vi "AplicaPond_C_Ref_GenExterno.vi"(1 "result":string[][](array[string])) -> (0 "output array":string[][](array[string]))   [LabVIEW 2019, in "Prueba03.lvclass"]
doc: "Aplica ponderacion C a la curva de referencia hecha en Ajustes Previos 3"
uses:
  Prueba03.lvclass
panel:
  out "114db(C)":string[](array[string])
  out "94db(C)":string[](array[string])
  # "Frecuencias"
  # "94dB"
  # "114dB"
  # "94dB(A)"
  # "114dB(A)"
  # "94dB(C)"
  # "114dB(C)"
  # "94dB(Z)"
  # "114dB(Z)"
  # "Correcciones Microfono"
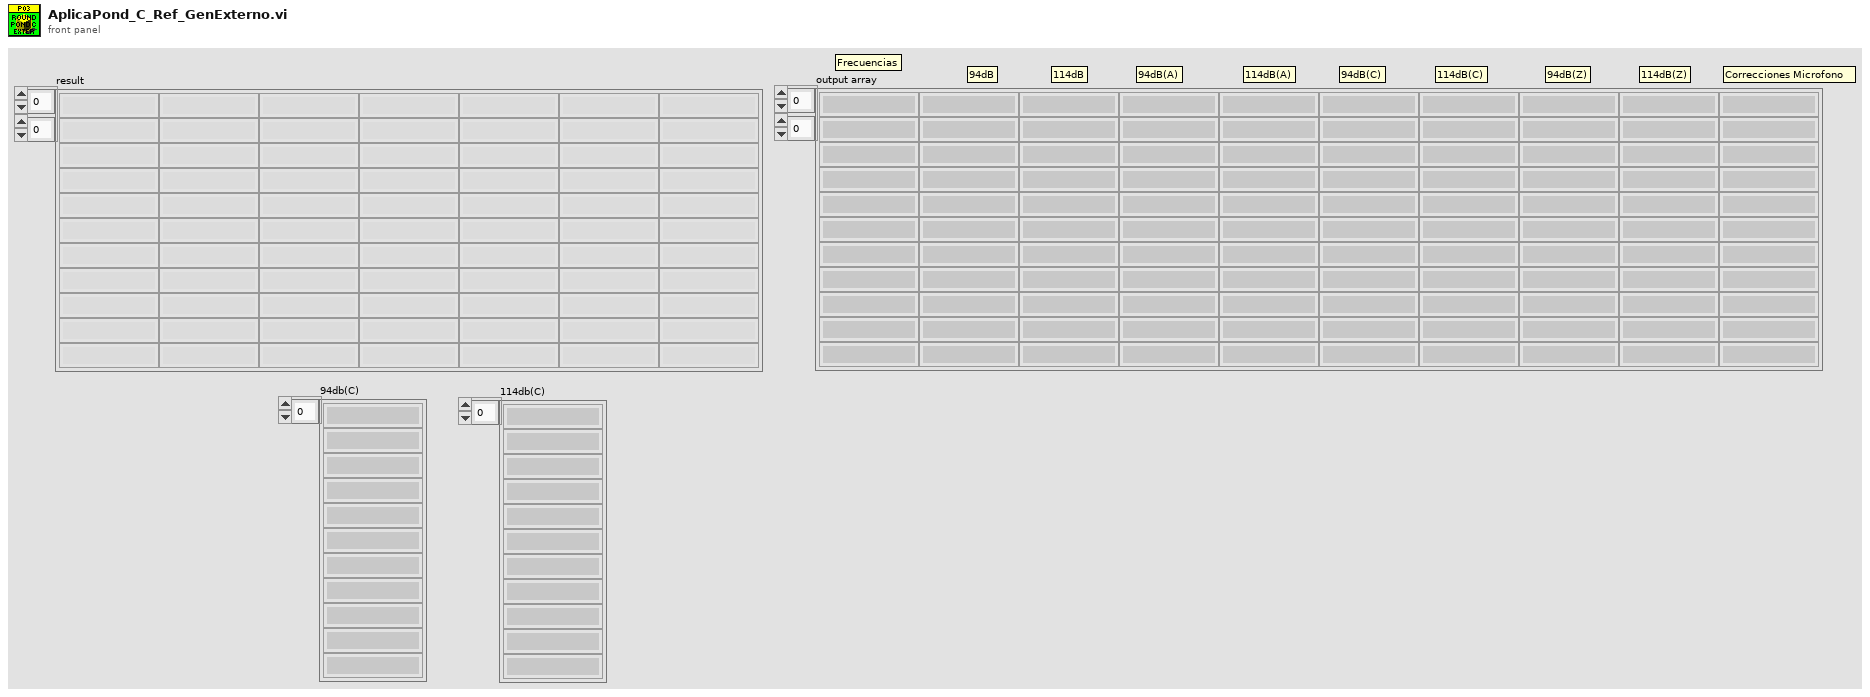
[diagram p1: front panel]
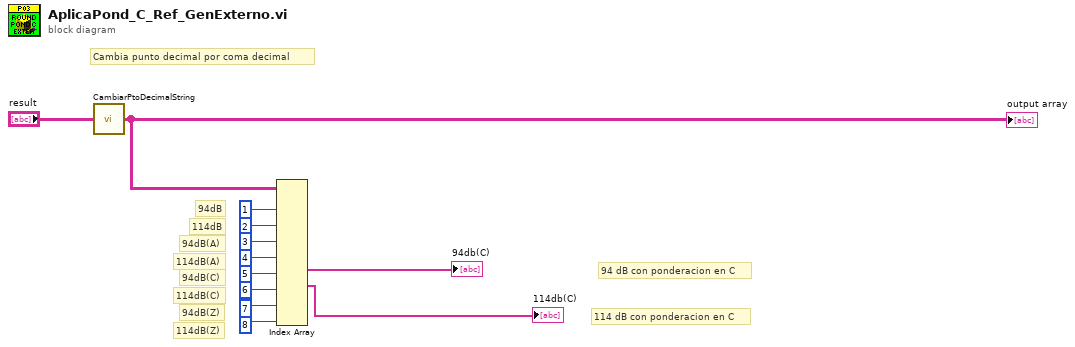
[diagram p0: block diagram]
diagram:
  # "114dB(Z)"
  # "94dB(Z)"
  # "114dB(C)"
  # "94dB(C)"
  # "114dB(A)"
  # "94dB(A)"
  # "114 dB con ponderacion en C"
  # "94 dB con ponderacion en C"
  # "114dB"
  # "94dB"
  # "Cambia punto decimal por coma decimal"
  n1 = call "CambiarPtoDecimalString.vi"("result"="result") -> ("result out"=w6:string[][])
  "output array" <- w6
  n2 = Index Array(array=w6, index (col) #1=1 ("disabled index (col)"), index (col) #2=2 ("disabled index (row)"), index (col) #3=3 ("index (col)"), index (col) #4=4 ("index (col)"), index (col) #5=5 ("index (col)"), index (col) #6=6 ("disabled index (row)"), index (col) #7=7 ("index (col)"), index (col) #8=8 ("index (col)")) -> (element #5=→"94db(C)":string[], element #6=→"114db(C)":string[])  [unwired: 8 in, 6 out]
